vi "parse key value pairs.vi"(10 "stream":string, 11 "dictionary in":variant) -> (3 "dictionary out":variant)   [LabVIEW 2013]
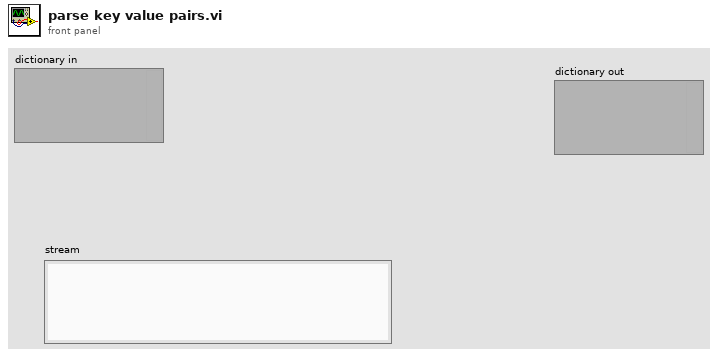
[diagram p1: front panel]
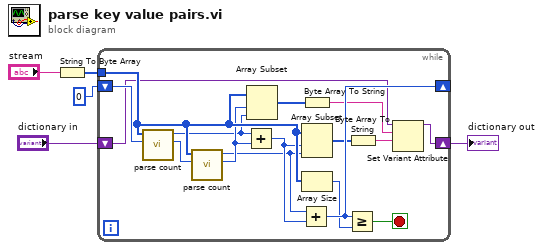
[diagram p0: block diagram]
diagram:
  n1 = String To Byte Array(string="stream") -> (unsigned byte array=w4:u8[])
  n2 = while {
    tunnel: w4 -> [w19]
    shift-right: [w18] -> _
    shift-left: 0 -> [w21]
    shift-right: [w8] -> w1
    shift-left: "dictionary in" -> [w9]
    stop <- w16 stop-if-true
    n3 = call "parse count.vi"("current index"=w21, "unsigned byte array"=w19) -> ("new index"=w20:i32, "count"=w13:u32)  [unwired: 8 in]
    n4 = call "parse count.vi"("current index"=w20, "unsigned byte array"=w19) -> ("new index"=w15:i32, "count"=w12:u32)  [unwired: 8 in]
    n5 = Add(x=w13, y=w15) -> (x+y=w14:u32)
    n6 = Array Subset(array=w19, index=w15, length=w13) -> (w11:u8[])
    n7 = Add(x=w12, y=w14) -> (x+y=w18:i32)
    n8 = Byte Array To String(unsigned byte array=w11) -> (string=w7:string)
    n9 = Array Subset(array=w19, index=w14, length=w12) -> (w10:u8[])
    n10 = Array Size(array=w19) -> (size(s)=w17:i32)
    n11 = Greater Or Equal?(x=w18, y=w17) -> (x >= y?=w16:bool)
    n12 = Byte Array To String(unsigned byte array=w10) -> (string=w6:string)
    n13 = Set Variant Attribute(Variant=w9, name=w7, value=w6) -> (Variant out=w8:variant)  [unwired: 1 in, 2 out]
  }
  "dictionary out" <- w1
